vi "Add Analog Output Channels.vi"(8 "error in (no error)":errorcluster, 9 "Analog Outputs":T1[](array[typedef]) {"ChannelType" items=["Voltage", "Current"]}, 11 "DAQ Ref":refnum<k24>) -> (0 "error out":errorcluster, 3 "DAQ Ref":refnum<k24>)   [LabVIEW 2019, in "Simple SysDef API.lvlib"]
uses:
  <userlib>/SimpleSysDef/Simple SysDef API.lvlib
  NationalInstruments.VeriStand.SystemDefinitionAPI
  <userlib>/SimpleSysDef/_SubVIs/Add DAQ Hardware_Analog Settings.ctl
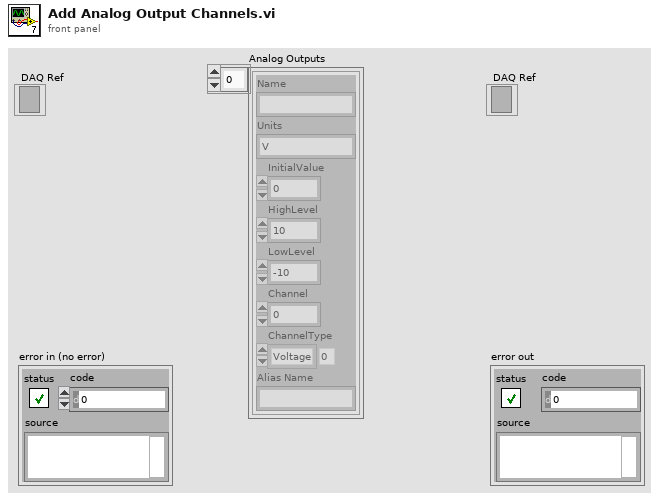
[diagram p1: front panel]
types:
  T1 = typedef "Simple SysDef API.lvlib/Add DAQ Hardware_Analog Settings.ctl" = cluster{"Name":string, "Units":string, "InitialValue":dbl, "HighLevel":dbl, "LowLevel":dbl, "Channel":u32, "ChannelType":i32, "Alias Name":string}
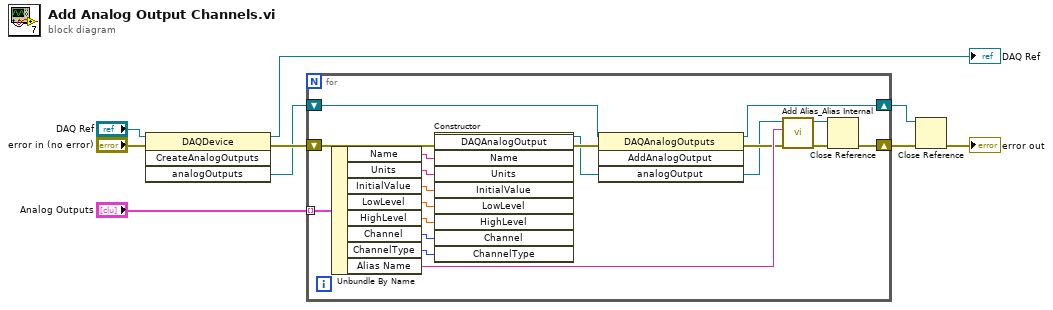
[diagram p0: block diagram]
diagram:
  n1 = invoke class="DAQDevice" method="CreateAnalogOutputs"(reference="DAQ Ref", error in="error in (no error)") -> (reference out=→"DAQ Ref":refnum<k24>, error out=w4:errorcluster, "analogOutputs"=w3:refnum<k24>)  [unwired: 2 in, 1 out]
  n2 = for {
    shift-right: [w24] -> w6
    shift-left: w4 -> [w26]
    tunnel: "Analog Outputs" -> [w22] mode=indexing
    shift-right: [w23] -> w7
    shift-left: w3 -> [w27]
    n3 = Unbundle By Name(w22) -> ("Name"=w21:string, "Units"=w20:string, "InitialValue"=w19:dbl, "LowLevel"=w18:dbl, "HighLevel"=w17:dbl, "Channel"=w16:u32, "ChannelType"=w15:i32, "Alias Name"=w14:string)
    n4 = constructor class="DAQAnalogOutput"(error in=w26, "Name"=w21, "Units"=w20, "InitialValue"=w19, "LowLevel"=w18, "HighLevel"=w17, "Channel"=w16, "ChannelType"=w15) -> (reference out=w11:refnum<k24>, error out=w25:errorcluster)  [unwired: 2 in, 8 out]
    n5 = invoke class="DAQAnalogOutputs" method="AddAnalogOutput"(reference=w27, error in=w25, "analogOutput"=w11) -> (reference out=w23:refnum<k24>, error out=w13:errorcluster)  [unwired: 1 in, 2 out]
    n6 = call <userlib>:"Add Alias_Alias Internal.vi"("error in (no error)"=w13, "Name"=w14, "Base Node"=w11) -> ("error out"=w12:errorcluster, "Base Node out"=w10:refnum<k24>)  [unwired: 7 in]
    n7 = Close Reference(reference=w10, error in (no error)=w12) -> (error out=w24:errorcluster)
  }
  n8 = Close Reference(reference=w7, error in (no error)=w6) -> (error out=→"error out":errorcluster)
